vi "Exame_3_Parte1.vi"() -> ()   [LabVIEW 2020]
panel:
  out "Valor Grafica":string
  out "Waveform Chart":i32(graph)
  in  "Cerrar":bool
  in  "Abrir":bool
  out "Pantalla":string
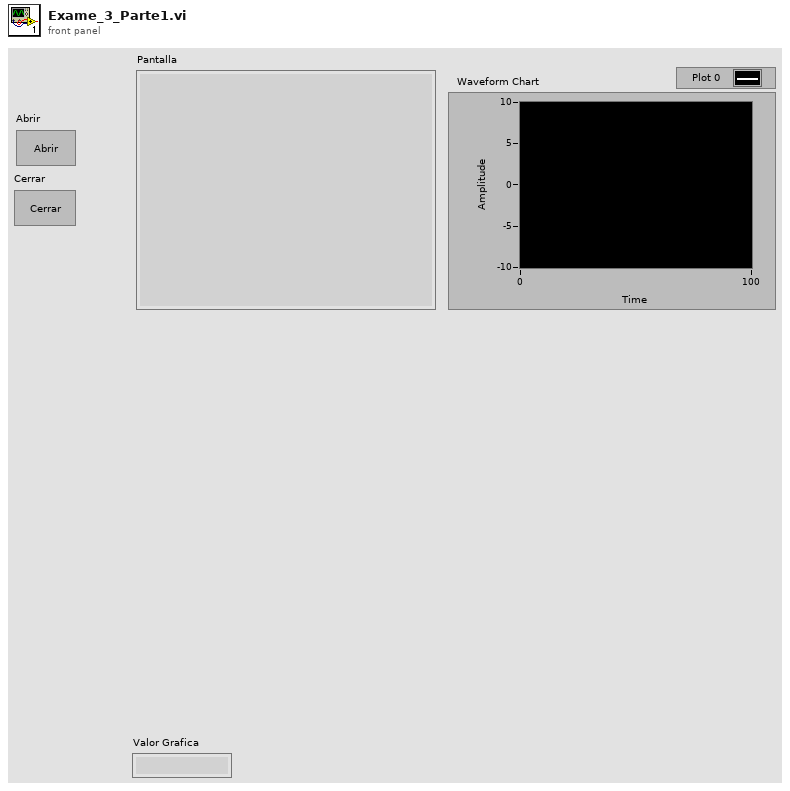
[diagram p1: front panel]
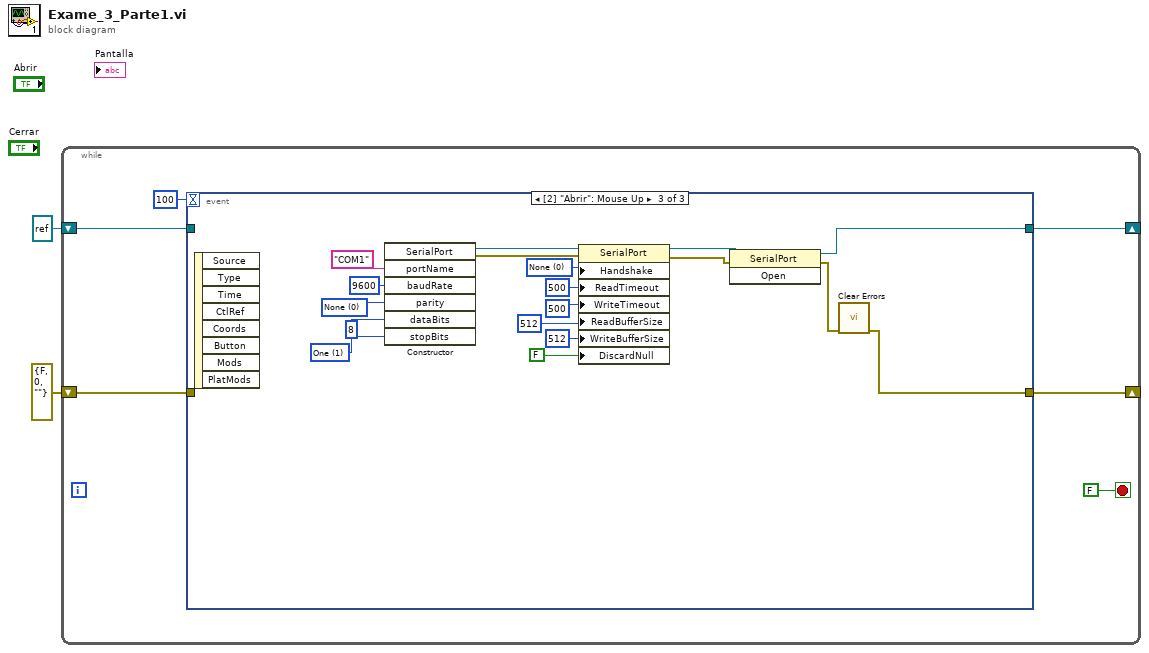
[diagram p0: block diagram]
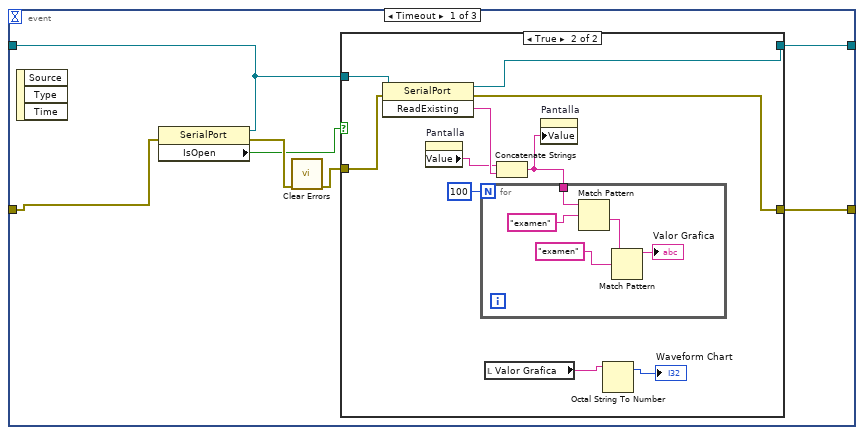
[diagram p2: hidden frame]
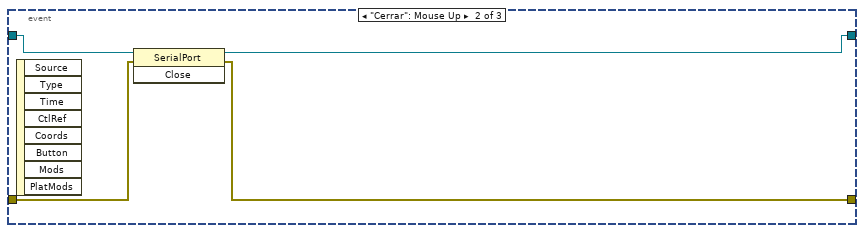
[diagram p4: hidden frame]
diagram:
  n1 = while {
    shift-right: [w7] -> _
    shift-left: refnum<k24> refnum ("SerialPort") -> [w5]
    shift-right: [w8] -> _
    shift-left: errorcluster {"status"=FALSE, "code"=0, "source"=""} ("error out") -> [w6]
    stop <- FALSE stop-if-true
    n2 = event shown="[2] \"Abrir\": Mouse Up" {
      selector: _ -> [_ _ _]
      dyn-events: _ -> [_ _ _]
      timeout: 100 -> [_ _ _]
      tunnel: [w15 w33 w38] -> w8
      tunnel: [w14 w34 w37] -> w7
      tunnel: w6 -> [w12 w35 _]
      tunnel: w5 -> [w13 w36 _]
      event Timeout {
        n3 = event-data() -> ()  [unwired: 1 in, 3 out]
        n4 = property class="SerialPort"(reference=w13, error in=w12) -> (error out=w11:errorcluster, "IsOpen"=w9:bool)  [unwired: 1 out]
        n5 = call <vilib>:"Clear Errors.vi"("error in (no error)"=w11) -> ("error out"=w10:errorcluster)  [unwired: 5 in, 1 out]
        n6 = case shown="True" w9 {
          tunnel: [w16 w27] -> w15
          tunnel: [w17 w26] -> w14
          tunnel: w13 -> [w17 w25]
          tunnel: w10 -> [w16 w24]
          frame False {
          }
          frame True {
            n7 = invoke class="SerialPort" method="ReadExisting"(reference=w25, error in=w24) -> (reference out=w26:refnum<k24>, error out=w27:errorcluster, "ReadExisting"=w23:string)  [unwired: 1 in]
            n8 = property on="Pantalla" class="Str"() -> ("Value"=w22:string)  [unwired: 2 in, 2 out]
            n9 = local read "Valor Grafica"() -> (w20:string)
            n10 = Concatenate Strings(w22, w23) -> (w21:string)
            n11 = for {
              N: 100 -> [_]
              tunnel: w21 -> [w32]
              n12 = Match Pattern(string=w32, regular expression="examen") -> (after substring=w29:string)  [unwired: 1 in, 3 out]
              n13 = Match Pattern(string=w29, regular expression="examen") -> (before substring=→"Valor Grafica":string)  [unwired: 1 in, 3 out]
            }
            n14 = property on="Pantalla" class="Str"("Value"=w21) -> ()  [unwired: 2 in, 2 out]
            n15 = Octal String To Number(4:w20) -> (1:→"Waveform Chart":i32)  [unwired: 2 in, 1 out]
          }
        }
      }
      event "Cerrar": Mouse Up {
        n16 = event-data() -> ()  [unwired: 1 in, 8 out]
        n17 = invoke class="SerialPort" method="Close"(reference=w36, error in=w35) -> (reference out=w34:refnum<k24>, error out=w33:errorcluster)  [unwired: 1 in, 1 out]
      }
      event "Abrir": Mouse Up {
        w49 = 0 items=["None", "XOnXOff", "RequestToSend", "RequestToSendXOnXOff"] ("Handshake")
        w39 = 1 items=["None", "One", "Two", "OnePointFive"] ("stopBits")
        w41 = 0 items=["None", "Odd", "Even", "Mark", "Space"] ("parity")
        n18 = event-data() -> ()  [unwired: 1 in, 8 out]
        n19 = constructor class="SerialPort"("portName"="COM1", "baudRate"=9600, "parity"=w41, "dataBits"=8, "stopBits"=w39) -> (error out=w50:errorcluster, "SerialPort"=w51:refnum<k24>)  [unwired: 3 in, 6 out]
        n20 = property class="SerialPort"(reference=w51, error in=w50, "Handshake"=w49, "ReadTimeout"=500, "WriteTimeout"=500, "ReadBufferSize"=512, "WriteBufferSize"=512, "DiscardNull"=FALSE) -> (reference out=w52:refnum<k24>, error out=w53:errorcluster)
        n21 = invoke class="SerialPort" method="Open"(reference=w52, error in=w53) -> (reference out=w37:refnum<k24>, error out=w54:errorcluster)  [unwired: 1 in, 1 out]
        n22 = call <vilib>:"Clear Errors.vi"("error in (no error)"=w54) -> ("error out"=w38:errorcluster)  [unwired: 5 in, 1 out]
      }
    }
  }
